vi "FTW-Panel-FrontPanel-SetVITitle.vi"(0 "Title":string, 1 "VI Refnum":refnum<vi>, 9 "Custom Title (T)":bool=TRUE, 11 "error in (no error)":errorcluster) -> (15 "error out":errorcluster)   [LabVIEW 2015]
doc: "Turns on the custom title for a VI and sets the text string. If a VI refnum is not passed, this will obtain and use the refnum of the calling VI.\n\nThe reference will not get closed if it is passed in. Suggest using <b>Get Parent VI Refnum.vi<b> if this is wrapped in an app specific VI."
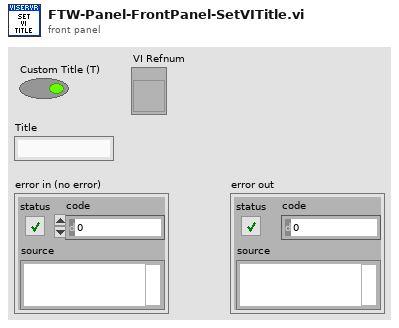
[diagram p1: front panel]
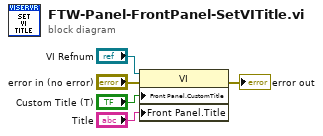
[diagram p0: block diagram]
diagram:
  n1 = property class="VI"(reference="VI Refnum", error in="error in (no error)", "Front Panel.CustomTitle"="Custom Title (T)", "Front Panel.Title"="Title") -> (error out=→"error out":errorcluster)  [unwired: 1 out]
